vi "Close.vi"(8 "error in (no error)":errorcluster, 11 "VICI Settings":T1) -> (0 "error out":errorcluster, 1 "Connection Error":bool, 3 "VICI Settings":T1)   [LabVIEW 2018, in "VICI M6 M50 Party Mode.lvlib"]
uses:
  VICI M6 M50 Party Mode.lvlib
  Settings Cluster.ctl
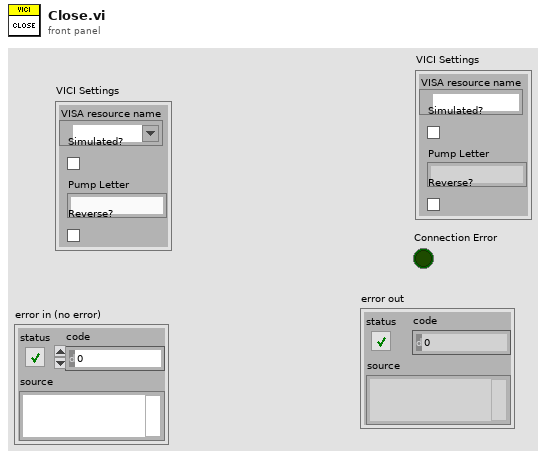
[diagram p1: front panel]
types:
  T1 = typedef "VICI M6 M50 Party Mode.lvlib/Settings Cluster.ctl" = cluster{"VISA resource name":refnum<visa-resource-name>, "Simulated?":bool, "Pump Letter":string, "Reverse?":bool}
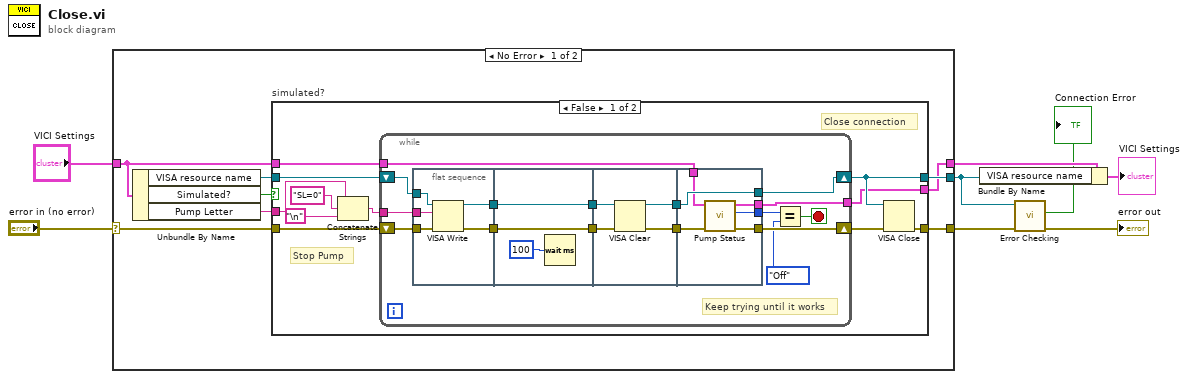
[diagram p0: block diagram]
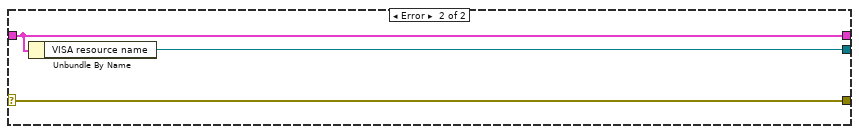
[diagram p3: hidden frame]
diagram:
  n1 = case shown="No Error" "error in (no error)" {
    selector: "error in (no error)" -> [w14 w67]
    tunnel: [w15 w67] -> w6
    tunnel: "VICI Settings" -> [w11 w65]
    tunnel: [w12 w66] -> w3
    tunnel: [w10 w65] -> w2
    frame No Error {
      n2 = Unbundle By Name(w11) -> ("VISA resource name"=w13:refnum<visa-resource-name>, "Simulated?"=w16:bool, "Pump Letter"=w9:string)
      n3 = case "simulated?" shown="False" w16 {
        tunnel: [w22 w64] -> w15
        tunnel: w13 -> [w21 w63]
        tunnel: w14 -> [w25 w64]
        tunnel: [w20 w63] -> w12
        tunnel: w11 -> [w19 w62]
        tunnel: [w18 w62] -> w10
        tunnel: w9 -> [w17 _]
        frame False {
          # "Close connection"
          # "Stop Pump"
          n4 = Concatenate Strings(w17, "SL=0" ("string"), "\n") -> (w24:string)
          n5 = while {
            tunnel: w24 -> [w36]
            shift-right: [w35] -> w23
            shift-left: w25 -> [w37]
            shift-right: [w33] -> w20
            shift-left: w21 -> [w34]
            tunnel: w19 -> [w31]
            tunnel: [w30] -> w18
            stop <- w32 stop-if-true
            # "Keep trying until it works"
            n6 = flat-sequence {
              tunnel: [w44] -> w43
              tunnel: [w45] -> w42
              tunnel: w37 -> [w48]
              tunnel: w36 -> [w47]
              tunnel: w34 -> [w46]
              tunnel: w43 -> [w51]
              tunnel: [w51] -> w41
              tunnel: w42 -> [w50]
              tunnel: [w50] -> w40
              tunnel: w41 -> [w55]
              tunnel: w40 -> [w54]
              tunnel: [w53] -> w39
              tunnel: [w52] -> w38
              tunnel: [w61] -> w33
              tunnel: [w59] -> w35
              tunnel: w39 -> [w60]
              tunnel: w38 -> [w61]
              tunnel: [w58] -> w29
              tunnel: w31 -> [w57]
              tunnel: [w56] -> w30
              frame #0 {
                n7 = VISA Write(VISA resource name=w46, write buffer=w47, error in (no error)=w48) -> (VISA resource name out=w44:refnum<visa-resource-name>, error out=w45:errorcluster)  [unwired: 1 out]
              }
              frame #1 {
                n8 = Wait (ms)(milliseconds to wait=u32 100) -> ()  [unwired: 1 out]
              }
              frame #2 {
                n9 = VISA Clear(VISA resource name=w55, error in (no error)=w54) -> (VISA resource name out=w52:refnum<visa-resource-name>, error out=w53:errorcluster)
              }
              frame #3 {
                n10 = call "Pump Status.vi"("error in (no error)"=w60, "VICI Settings"=w57) -> ("error out"=w59:errorcluster, "Pump On?"=w58:enum16{"Off", "On", "Not Initialized"}, "VICI Settings"=w56:T1)  [unwired: 6 in, 1 out]
              }
            }
            n11 = Equal?(x=w29, y=enum16{"Off", "On", "Not Initialized"}."Off") -> (x = y?=w32:bool)
          }
          n12 = VISA Close(VISA resource name=w20, error in (no error)=w23) -> (error out=w22:errorcluster)
        }
        frame True {
        }
      }
    }
    frame Error {
      n13 = Unbundle By Name(w65) -> ("VISA resource name"=w66:refnum<visa-resource-name>)
    }
  }
  n14 = Bundle By Name(cluster=w2, "VISA resource name"=w3) -> (→"VICI Settings":T1)
  n15 = call "Error Checking.vi"("error in (no error)"=w6, "VISA resource name"=w3) -> ("error out"=→"error out":errorcluster, "Connection Error"=→"Connection Error":bool)  [unwired: 7 in, 1 out]
